vi "Apply Arc Velocity to Motors.vi"(6 "constraint error tolerance (1E-12)":dbl=1e-12, 7 "wheel indexes":i32[](array[numeric]), 8 "error in (no error)":errorcluster, 10 "arc velocity":T1={"turning radius"=1.0, "tangential velocity"=0.0, "angle from tangent (rad)"=0.0}, 11 "steering frame in":refnum<class "NI_Robotics_Steering Frame.lvclass">) -> (0 "error out":errorcluster, 1 "ccw motor angle setpoints (rad)":dbl[](array[numeric]), 2 "ccw motor velocity setpoints":dbl[](array[numeric]), 3 "steering frame out":refnum<class "NI_Robotics_Steering Frame.lvclass">, 4 "ccw caster motor velocity setpoints":dbl[](array[numeric]))   [LabVIEW 2017, in "NI_Robotics_Steering Frame.lvclass"]
doc: "Calculates the velocity and angle of each motor necessary to satisfy the <B>steering frame velocity</B> or <B>arc velocity</B> at the center of a steering frame. You must manually select the polymorphic instance to use."
uses:
  <vilib>/robotics/Steering/Steering Frame/NI_Robotics_Steering Frame.lvclass
  <vilib>/robotics/Steering/Steering Frame/Arc Velocity.ctl
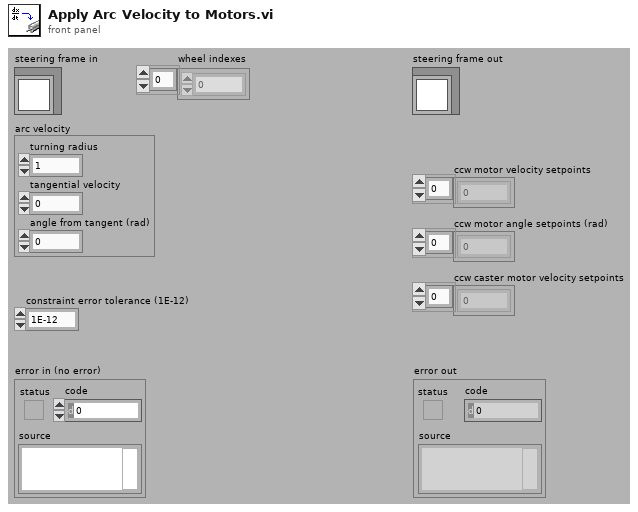
[diagram p1: front panel]
types:
  T1 = typedef "NI_Robotics_Steering Frame.lvclass/Arc Velocity.ctl" = cluster{"turning radius":dbl, "tangential velocity":dbl, "angle from tangent (rad)":dbl}
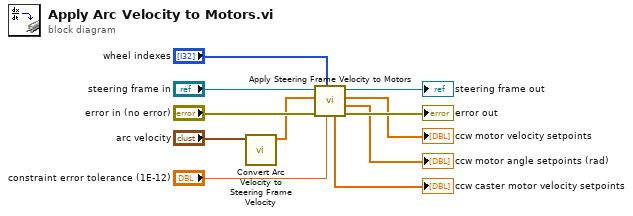
[diagram p0: block diagram]
diagram:
  n1 = call <vilib>:"Convert Arc Velocity to Steering Frame Velocity.vi"("arc velocity"="arc velocity") -> ("steering frame velocity"=w1:dbl[])  [unwired: 10 in]
  n2 = call <vilib>:"Apply Steering Frame Velocity to Motors.vi"("constraint error tolerance (1E-12)"="constraint error tolerance (1E-12)", "wheel indexes"="wheel indexes", "error in (no error)"="error in (no error)", "steering frame velocity"=w1, "steering frame in"="steering frame in") -> ("error out"=→"error out":errorcluster, "ccw motor angle setpoints (rad)"=→"ccw motor angle setpoints (rad)":dbl[], "ccw motor velocity setpoints"=→"ccw motor velocity setpoints":dbl[], "steering frame out"=→"steering frame out":refnum<class "NI_Robotics_Steering Frame.lvclass">, "ccw caster motor velocity setpoints"=→"ccw caster motor velocity setpoints":dbl[])  [unwired: 2 in]
